vi "Parse Date String.vi"(8 "error in":errorcluster, 11 "Date String":string) -> (0 "error out":errorcluster, 3 "Time Stamp":timestamp format="%<%m/%d/%Y %H:%M:%S>T")   [LabVIEW 2020, in "Peer Review.lvclass"]
uses:
  Peer Review.lvclass
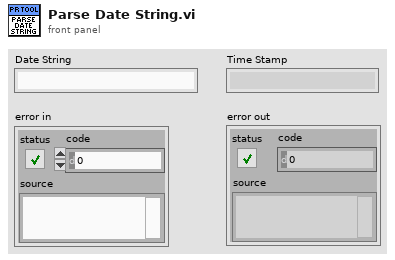
[diagram p1: front panel]
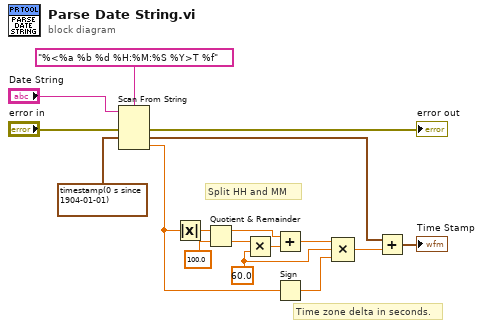
[diagram p0: block diagram]
diagram:
  w2 = 60.0 ("y")
  # "Time zone delta in seconds."
  # "Split HH and MM"
  n1 = Scan From String(format string="%<%a %b %d %H:%M:%S %Y>T %f", input string="Date String", error in="error in", default 1=timestamp(0 s since 1904-01-01)) -> (error out=→"error out":errorcluster, output 1=w11:timestamp, output 2=w6:dbl)  [unwired: 2 in, 2 out]
  n2 = Absolute Value(x=w6) -> (abs(x)=w7:dbl)
  n3 = Quotient & Remainder(x=w7, y=100.0) -> (x-y*floor(x/y)=w12:dbl, floor(x/y)=w13:dbl)
  n4 = Multiply(x=w13, y=w2) -> (x*y=w5:dbl)
  n5 = Add(x=w12, y=w5) -> (x+y=w4:dbl)
  n6 = Sign(1:w6) -> (0:w3:dbl)
  n7 = Compound Arithmetic op=MULTIPLY(w4, w2, w3) -> (w9:dbl)
  n8 = Add(x=w11, y=w9) -> (x+y=→"Time Stamp":timestamp)
